vi "Read Verbose.vi"(8 "error in (no error)":errorcluster, 11 "Test Manager":refnum<class "Test Manager.lvclass">) -> (0 "error out":errorcluster, 2 "Verbose":bool, 3 "Test Manager":refnum<class "Test Manager.lvclass">)   [LabVIEW 2013, in "Caraya.lvlib" / "Test Manager.lvclass"]
uses:
  Test Manager/Test Manager.lvclass
  Test Manager/Test Manager.lvclass/Test Manager.ctl
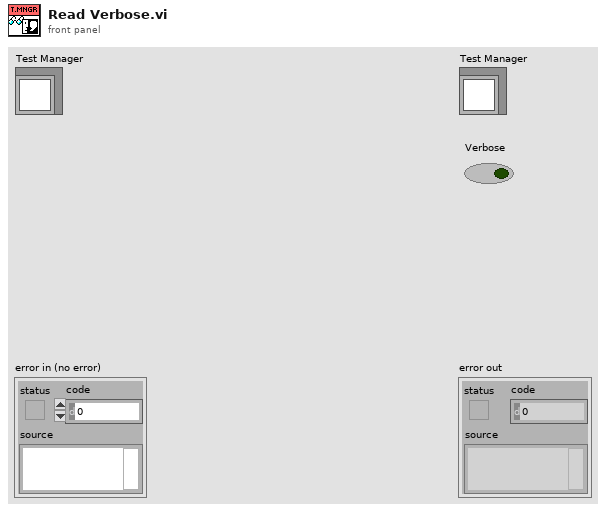
[diagram p1: front panel]
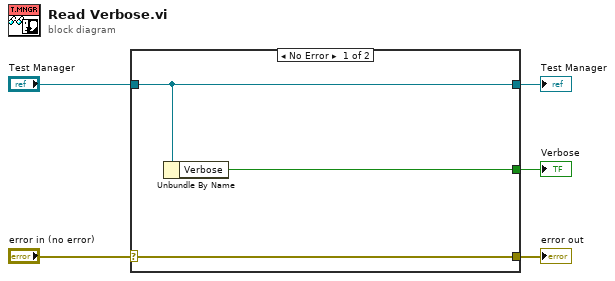
[diagram p0: block diagram]
diagram:
  n1 = case shown="No Error" "error in (no error)" {
    selector: "error in (no error)" -> [w8 w9]
    tunnel: [w8 w9] -> w4
    tunnel: [w7 w10] -> w2
    tunnel: "Test Manager" -> [w7 w10]
    tunnel: [w6 _] -> w1
    frame No Error {
      n2 = Unbundle By Name(w7) -> ("Verbose"=w6:bool)
    }
    frame Error {
    }
  }
  "error out" <- w4
  "Test Manager" <- w2
  "Verbose" <- w1
